vi "Example Threshold - OzoneConcentrationReached Callback.vi"(4 "OzoneConcentrationReached":refnum<user-event>, 5 "Event Data":T1, 6 "Control Ref":refnum<k24>, 7 "Event Common Data":T2) -> ()   [LabVIEW 2013]
uses:
  C:/tf/play/labview/Tinkerforge.dll
  Tinkerforge.dll
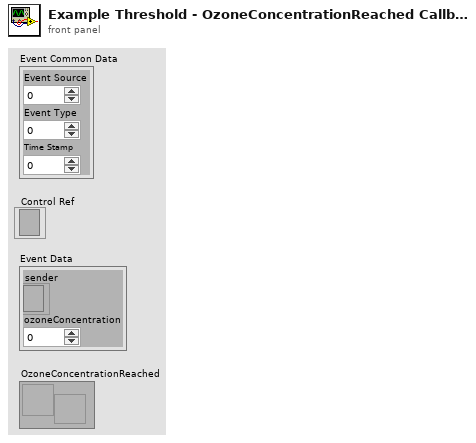
[diagram p1: front panel]
types:
  T1 = cluster{"sender":refnum<k24>, "ozoneConcentration":i32}
  T2 = cluster{"Event Source":i32, "Event Type":u32, "Time Stamp":u32}
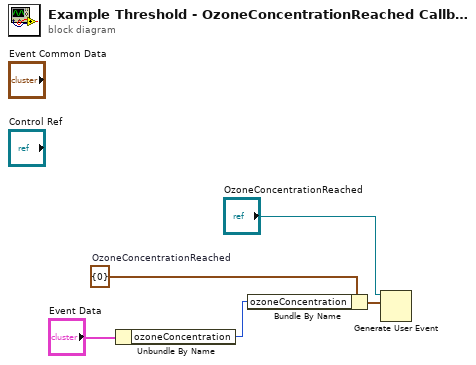
[diagram p0: block diagram]
diagram:
  w5 = cluster{"ozoneConcentration":i32} {"ozoneConcentration"=0}  # OzoneConcentrationReached
  n1 = Unbundle By Name("Event Data") -> ("ozoneConcentration"=w3:i32)
  n2 = Bundle By Name(cluster=w5, "ozoneConcentration"=w3) -> (w2:cluster{"ozoneConcentration":i32})
  n3 = Generate User Event(user event="OzoneConcentrationReached", event data cluster=w2) -> ()  [unwired: 2 in, 2 out]
